vi "Test Compare Equal 8bit Enums.vi"(8 "error in (no error)":errorcluster, 11 "Comparison Test Double in":refnum<class "Comparison Test Double.lvclass">) -> (0 "error out":errorcluster, 3 "Comparison Test Double out":refnum<class "Comparison Test Double.lvclass">)   [LabVIEW 2020, in "Comparison Test Double.lvclass"]
uses:
  Comparison Test Double.lvclass
  C:/git/astemes-lunit/source/LUnit Test Case.lvclass
  source/LUnit Test Case.lvclass/LUnit Test Case.ctl
  23615402-9b1f-4bd5-97a8-ca362d09ae43.vi
  source/Core/LUnit Test Case/Private/Append Pass Result.vi
  source/Core/LUnit Test Case/Private/Append Fail Result.vi
  23615402-9b1f-4bd5-97a8-ca362d09ae43.vi/9c5d11cd-9439-4240-a1ee-d9baace9c924.vi
  source/Core/LUnit Test Case/Private/Run In UI.vi
  <vilib>/Utility/error.llb/Clear Errors.vi
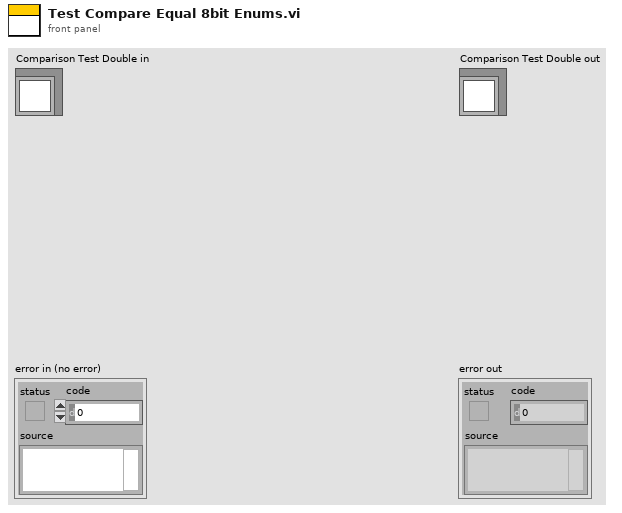
[diagram p1: front panel]
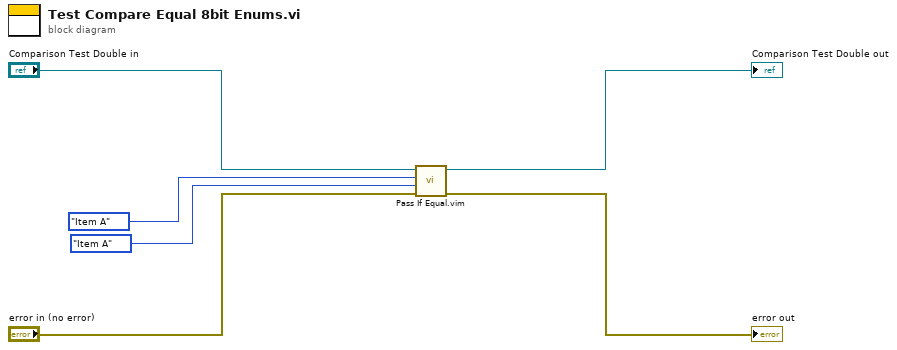
[diagram p0: block diagram]
diagram:
  n1 = call "Pass If Equal.vim"("error in (no error)"="error in (no error)", "Actual"=enum8{"Item A", "Item B"}."Item A", "Expected"=enum8{"Item A", "Item B"}."Item A", "LUnit Test Case In"="Comparison Test Double in") -> ("error out"=→"error out":errorcluster, "LUnit Test Case Out"=→"Comparison Test Double out":refnum<class "Comparison Test Double.lvclass">)  [unwired: 6 in]
